vi "CreatePrivateEvents.vi"(8 "error in (no error)":errorcluster, 11 "Setting Database":refnum<class "Setting Database.lvclass">) -> (0 "error out":errorcluster, 3 "Setting Database out":refnum<class "Setting Database.lvclass">)   [LabVIEW 2019, in "Setting Database.lvclass"]
doc: "---------------------------------------------------------------\nJKI State Machine Objects™\nhttp://jki.net/state-machine-objects/\nCopyright (C) 2005-2015, JKI <info@jki.net>\nALL RIGHTS RESERVEDJKI State Machine Objects (SMO) 1.0.0.4\nJKI - JKI\nCopyright (c) 2015, JKI"
uses:
  Setting Database.lvclass
  Typedefs/PrivateEvents--Setting Database.SetActivePath.ctl
  Typedefs/PrivateEvents--Setting Database.UpdateActivePath.ctl
  Path Settings/Path Settings.lvclass
  Typedefs/PrivateEvents--Setting Database.Refresh.ctl
  Typedefs/PrivateEvents--Setting Database.CopyActivePathToAll.ctl
  Typedefs/PrivateEvents--Setting Database.SetActiveRectangle.ctl
  Typedefs/PrivateEvents--Setting Database.UpdateActiveRectangle.ctl
  Rectangle Settings/Rectangle Settings.lvclass
  Typedefs/PrivateEvents--Setting Database.CopyActiveRectangleToAll.ctl
  Typedefs/PrivateEvents--Setting Database.SetActiveFunnel.ctl
  Typedefs/PrivateEvents--Setting Database.UpdateActiveFunnel.ctl
  Funnel Settings/Funnel Settings.lvclass
  Typedefs/PrivateEvents--Setting Database.CopyActiveFunnelToAll.ctl
  Typedefs/PrivateEvents--Setting Database.SetDefaultPath.ctl
  Typedefs/PrivateEvents--Setting Database.SetDefaultRectangle.ctl
  Typedefs/PrivateEvents--Setting Database.SetDefaultFunnel.ctl
  Typedefs/PrivateEvents--Setting Database.SetDefaultDot.ctl
  Typedefs/PrivateEvents--Setting Database.SetActiveDot.ctl
  Typedefs/PrivateEvents--Setting Database.UpdateActiveDot.ctl
  Dot Settings/Dot Settings.lvclass
  Typedefs/PrivateEvents--Setting Database.CopyActiveDotToAll.ctl
  Typedefs/PrivateEvents--Setting Database.ChangeObjectEnable.ctl
  Setting Database.lvclass/Setting Database.ctl
  <vilib>/JKI/JKI SMO/SMO/SMO.lvclass
panel:
  # "For instructions on how to use the JKI State Machine Objects, examples and video tutorials, visit:\nhttp://jki.net/state-machine-objects/\n\nJKI State Machine Objects™\nhttp://jki.net/state-machine-objects/\nCopyright (C) 2005-2015, JKI <info@jki.net>\nALL RIGHTS RESERVED"
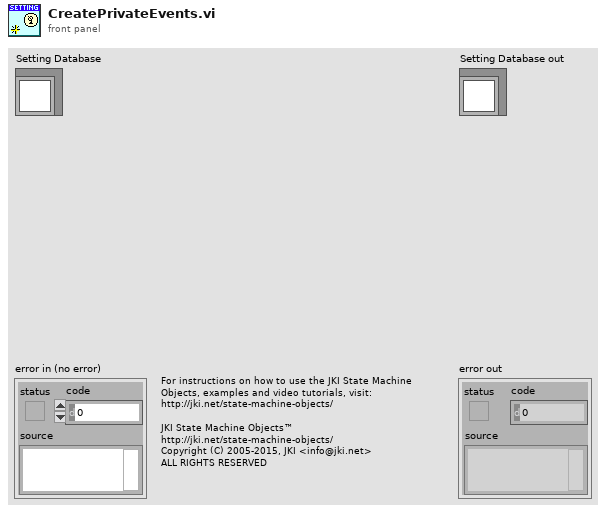
[diagram p1: front panel]
types:
  T1 = typedef "Setting Database.lvclass/PrivateEvents--Setting Database.ChangeObjectEnable.ctl" = string
  T2 = typedef "Setting Database.lvclass/PrivateEvents--Setting Database.CopyActiveDotToAll.ctl" = bool
  T3 = typedef "Setting Database.lvclass/PrivateEvents--Setting Database.UpdateActiveDot.ctl" = refnum<class "Dot Settings.lvclass">
  T4 = typedef "Setting Database.lvclass/PrivateEvents--Setting Database.SetActiveDot.ctl" = i32
  T5 = typedef "Setting Database.lvclass/PrivateEvents--Setting Database.SetDefaultDot.ctl" = bool
  T6 = typedef "Setting Database.lvclass/PrivateEvents--Setting Database.SetDefaultFunnel.ctl" = bool
  T7 = typedef "Setting Database.lvclass/PrivateEvents--Setting Database.SetDefaultRectangle.ctl" = bool
  T8 = typedef "Setting Database.lvclass/PrivateEvents--Setting Database.SetDefaultPath.ctl" = bool
  T9 = typedef "Setting Database.lvclass/PrivateEvents--Setting Database.CopyActiveFunnelToAll.ctl" = bool
  T10 = typedef "Setting Database.lvclass/PrivateEvents--Setting Database.UpdateActiveFunnel.ctl" = refnum<class "Funnel Settings.lvclass">
  T11 = typedef "Setting Database.lvclass/PrivateEvents--Setting Database.SetActiveFunnel.ctl" = i32
  T12 = typedef "Setting Database.lvclass/PrivateEvents--Setting Database.CopyActiveRectangleToAll.ctl" = bool
  T13 = typedef "Setting Database.lvclass/PrivateEvents--Setting Database.UpdateActiveRectangle.ctl" = refnum<class "Rectangle Settings.lvclass">
  T14 = typedef "Setting Database.lvclass/PrivateEvents--Setting Database.SetActiveRectangle.ctl" = i32
  T15 = typedef "Setting Database.lvclass/PrivateEvents--Setting Database.CopyActivePathToAll.ctl" = bool
  T16 = typedef "Setting Database.lvclass/PrivateEvents--Setting Database.Refresh.ctl" = cluster{"Paths":i32, "Rectangles":i32, "Funnels":i32, "Dots":i32}
  T17 = typedef "Setting Database.lvclass/PrivateEvents--Setting Database.UpdateActivePath.ctl" = refnum<class "Path Settings.lvclass">
  T18 = typedef "Setting Database.lvclass/PrivateEvents--Setting Database.SetActivePath.ctl" = i32
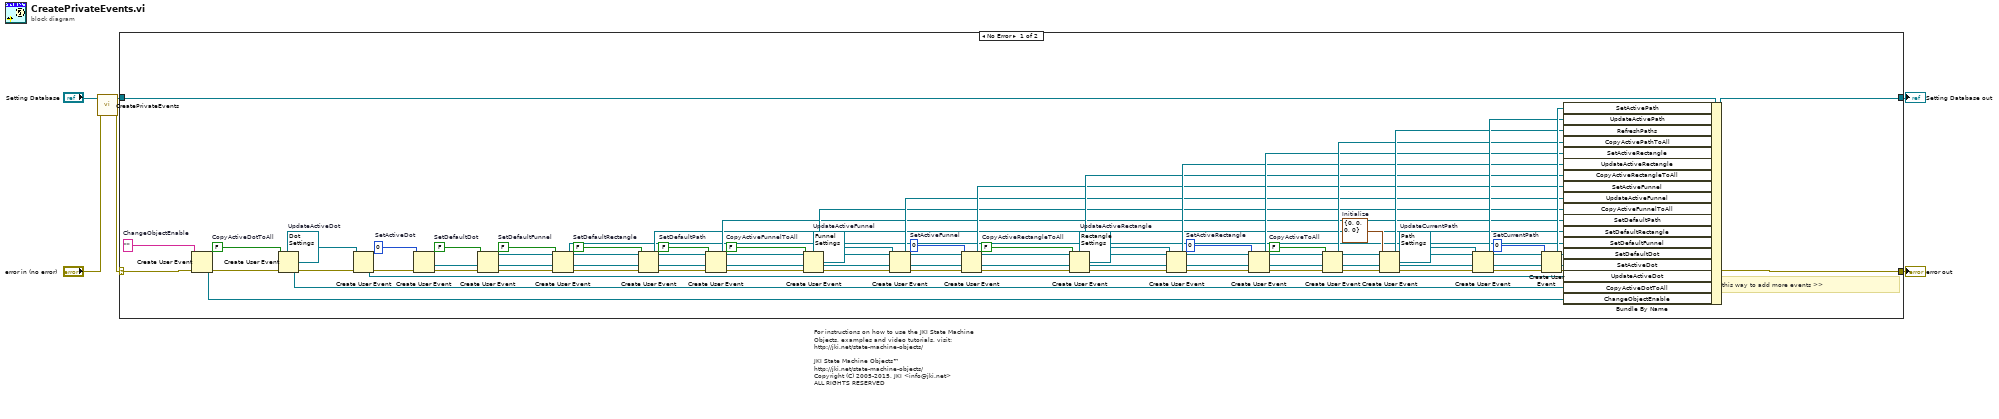
[diagram p0: block diagram]
diagram:
  # "For instructions on how to use the JKI State Machine Objects, examples and video tutorials, visit:\nhttp://jki.net/state-machine-objects/\n\nJKI State Machine Objects™\nhttp://jki.net/state-machine-objects/\nCopyright (C) 2005-2015, JKI <info@jki.net>\nALL RIGHTS RESERVED"
  n1 = call-parent "CreatePrivateEvents.vi"("error in (no error)"="error in (no error)", "SMO"="Setting Database") -> ("error out"=w1:errorcluster, "SMO out"=w3:refnum<class "Setting Database.lvclass">)  [unwired: 8 in]
  n2 = case shown="No Error" w1 {
    selector: w1 -> [w62 w65]
    tunnel: [w60 w65] -> w5
    tunnel: [w61 w64] -> w6
    tunnel: w3 -> [w63 w64]
    frame No Error {
      w8 = T1 ""  # ChangeObjectEnable
      w11 = T2 FALSE  # CopyActiveDotToAll
      w14 = T3 refnum  # UpdateActiveDot
      w17 = T4 0  # SetActiveDot
      w20 = T5 FALSE  # SetDefaultDot
      w23 = T6 FALSE  # SetDefaultFunnel
      w26 = T7 FALSE  # SetDefaultRectangle
      w29 = T8 FALSE  # SetDefaultPath
      w32 = T9 FALSE  # CopyActiveFunnelToAll
      w35 = T10 refnum  # UpdateActiveFunnel
      w38 = T11 0  # SetActiveFunnel
      w41 = T12 FALSE  # CopyActiveRectangleToAll
      w44 = T13 refnum  # UpdateActiveRectangle
      w47 = T14 0  # SetActiveRectangle
      w50 = T15 FALSE  # CopyActiveToAll
      w53 = T16 {"Paths"=0, "Rectangles"=0, "Funnels"=0, "Dots"=0}  # Initialize
      w56 = T17 refnum  # UpdateCurrentPath
      w59 = T18 0  # SetCurrentPath
      # "Expand this way to add more events >>"
      n3 = Create User Event(user event datatype=w8, error in=w62) -> (user event=w7:refnum<user-event>, error out=w9:errorcluster)
      n4 = Create User Event(user event datatype=w11, error in=w9) -> (user event=w10:refnum<user-event>, error out=w12:errorcluster)
      n5 = Create User Event(user event datatype=w14, error in=w12) -> (user event=w13:refnum<user-event>, error out=w15:errorcluster)
      n6 = Create User Event(user event datatype=w17, error in=w15) -> (user event=w16:refnum<user-event>, error out=w18:errorcluster)
      n7 = Create User Event(user event datatype=w20, error in=w18) -> (user event=w19:refnum<user-event>, error out=w21:errorcluster)
      n8 = Create User Event(user event datatype=w23, error in=w21) -> (user event=w22:refnum<user-event>, error out=w24:errorcluster)
      n9 = Create User Event(user event datatype=w26, error in=w24) -> (user event=w25:refnum<user-event>, error out=w27:errorcluster)
      n10 = Create User Event(user event datatype=w29, error in=w27) -> (user event=w28:refnum<user-event>, error out=w30:errorcluster)
      n11 = Create User Event(user event datatype=w32, error in=w30) -> (user event=w31:refnum<user-event>, error out=w33:errorcluster)
      n12 = Create User Event(user event datatype=w35, error in=w33) -> (user event=w34:refnum<user-event>, error out=w36:errorcluster)
      n13 = Create User Event(user event datatype=w38, error in=w36) -> (user event=w37:refnum<user-event>, error out=w39:errorcluster)
      n14 = Create User Event(user event datatype=w41, error in=w39) -> (user event=w40:refnum<user-event>, error out=w42:errorcluster)
      n15 = Create User Event(user event datatype=w44, error in=w42) -> (user event=w43:refnum<user-event>, error out=w45:errorcluster)
      n16 = Create User Event(user event datatype=w47, error in=w45) -> (user event=w46:refnum<user-event>, error out=w48:errorcluster)
      n17 = Create User Event(user event datatype=w50, error in=w48) -> (user event=w49:refnum<user-event>, error out=w51:errorcluster)
      n18 = Create User Event(user event datatype=w53, error in=w51) -> (user event=w52:refnum<user-event>, error out=w54:errorcluster)
      n19 = Create User Event(user event datatype=w56, error in=w54) -> (user event=w55:refnum<user-event>, error out=w57:errorcluster)
      n20 = Create User Event(user event datatype=w59, error in=w57) -> (user event=w58:refnum<user-event>, error out=w60:errorcluster)
      n21 = Bundle By Name(cluster=w63, "SetActivePath"=w58, "UpdateActivePath"=w55, "RefreshPaths"=w52, "CopyActivePathToAll"=w49, "SetActiveRectangle"=w46, "UpdateActiveRectangle"=w43, "CopyActiveRectangleToAll"=w40, "SetActiveFunnel"=w37, "UpdateActiveFunnel"=w34, "CopyActiveFunnelToAll"=w31, "SetDefaultPath"=w28, "SetDefaultRectangle"=w25, "SetDefaultFunnel"=w22, "SetDefaultDot"=w19, "SetActiveDot"=w16, "UpdateActiveDot"=w13, "CopyActiveDotToAll"=w10, "ChangeObjectEnable"=w7) -> (w61:refnum<class "Setting Database.lvclass">)
    }
    frame Error {
    }
  }
  "error out" <- w5
  "Setting Database out" <- w6
